vi "Add Labels.vi"(6 "Variant in":variant, 7 "Shift Pressed?":bool, 8 "error in (no error)":errorcluster, 10 "QD Combo Box Ref":refnum<vi>, 11 "QD Launch VI Ref":refnum<vi>) -> (0 "error out":errorcluster, 4 "Variant out":variant)   [LabVIEW 2017]
doc: "Add labels to SubVIs, labels to structure objects or wire labels.\n\nUsage:\nThis quick-drop plug-in works only in the block diagram.\nPress Ctrl+Space Ctrl+Q to add the labels to the selected items. If you insert a text into the combo box you will add this to the wire label.\nIf the plug-in is called using the SHIFT key than the label will be removed. \n\nDefault Shortcut - [Q]"
uses:
  8d00bab7-6807-40e1-91ac-73bbb8bf2eb0.vi
  78b8683c-1840-4b62-98b6-1b9e21eee10c.vi
panel:
  # "Do not change the connector pane of this VI.\n\nSee the block diagram for directions on how to use this template."
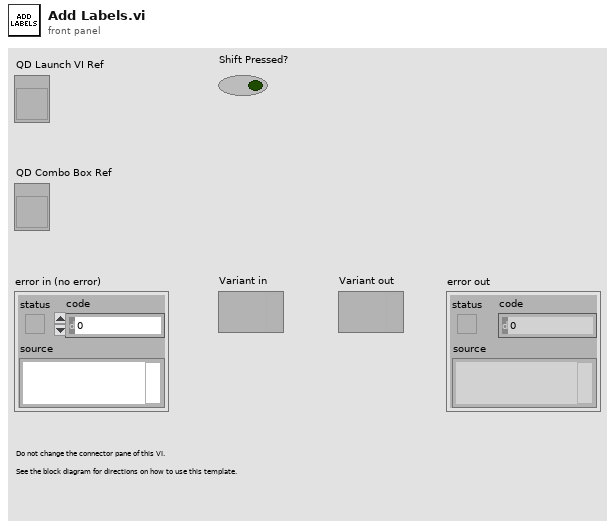
[diagram p1: front panel]
types:
  T1 = enum16{"MultiFrameStructure", "Structure", "Wire", "Constant", "FlatSequence", "Node"}
  T2 = enum16{"MultiFrameStructure", "Structure", "Wire", "Constant", "FlatSequence", "Node"}[]
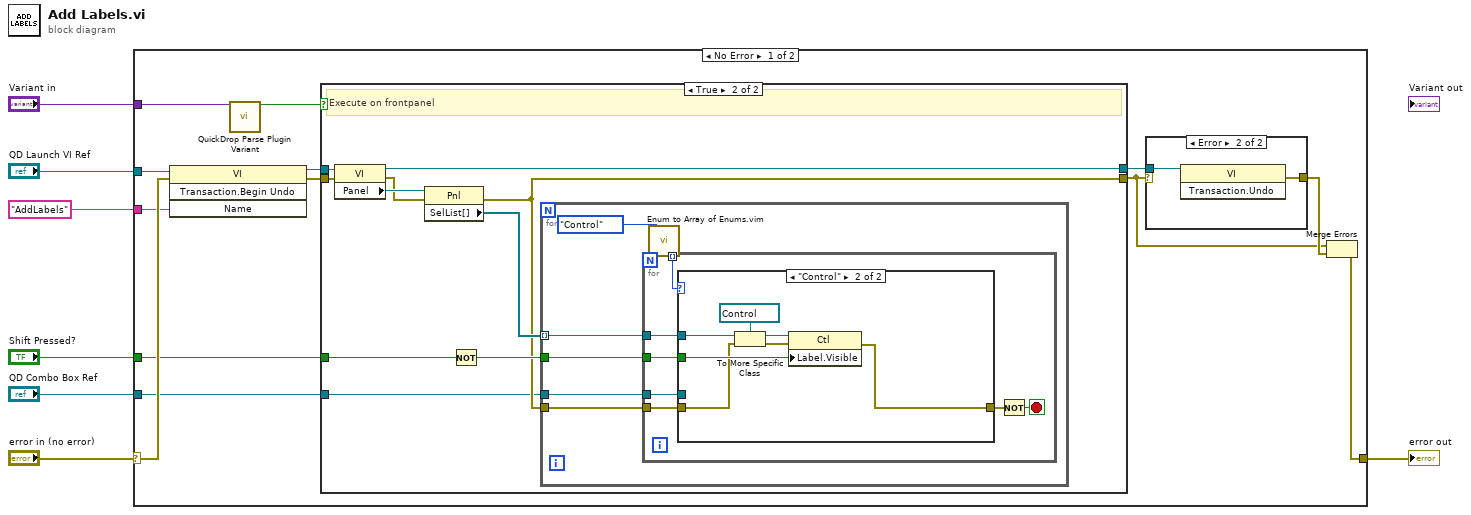
[diagram p0: block diagram]
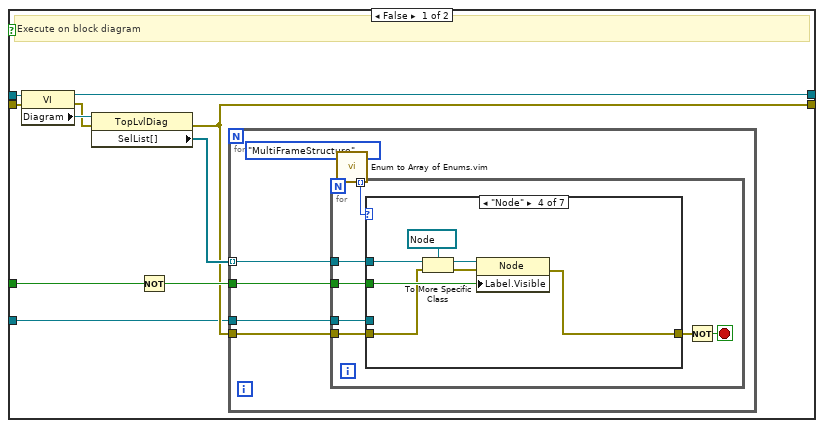
[diagram p2: hidden frame]
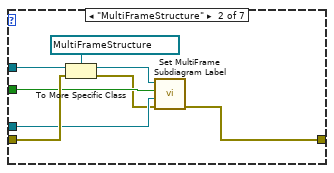
[diagram p4: hidden frame]
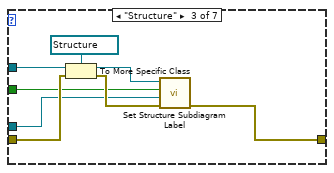
[diagram p5: hidden frame]
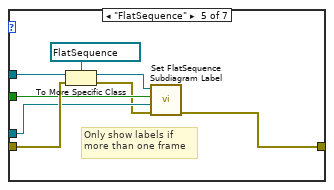
[diagram p6: hidden frame]
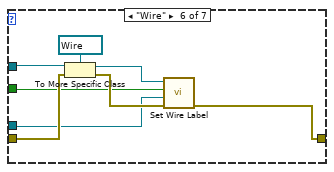
[diagram p7: hidden frame]
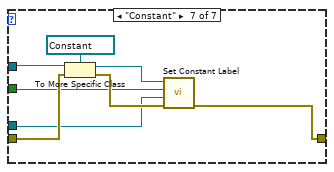
[diagram p8: hidden frame]
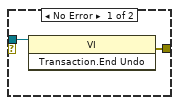
[diagram p10: hidden frame]
diagram:
  n1 = case shown="No Error" "error in (no error)" {
    selector: "error in (no error)" -> [w19 w127]
    tunnel: [w9 w127] -> w2
    tunnel: "Variant in" -> [w20 _]
    tunnel: "QD Launch VI Ref" -> [w17 _]
    tunnel: "AddLabels" ("Undo Name") -> [w18 _]
    tunnel: "Shift Pressed?" -> [w11 _]
    tunnel: "QD Combo Box Ref" -> [w10 _]
    frame No Error {
      n2 = invoke class="VI" method="Transaction.Begin Undo"(reference=w17, error in=w19, "Name"=w18) -> (reference out=w14:refnum<vi>, error out=w15:errorcluster)  [unwired: 1 in, 2 out]
      n3 = call <vilib>:"QuickDrop Parse Plugin Variant.vi"("QDKS Variant in"=w20) -> ("QD Launch VI Panel?"=w13:bool)  [unwired: 12 in, 2 out]
      n4 = case shown="True" w13 {
        tunnel: w15 -> [w30 w101]
        tunnel: w14 -> [w29 w100]
        tunnel: [w23 w94] -> w8
        tunnel: [w25 w96] -> w12
        tunnel: w11 -> [w21 w92]
        tunnel: w10 -> [w22 w93]
        frame False {
          # "Execute on block diagram"
          n5 = property class="VI"(reference=w29, error in=w30) -> (reference out=w25:refnum<vi>, error out=w26:errorcluster, "Diagram"=w28:refnum<vi>)
          n6 = property class="TopLvlDiag"(reference=w28, error in=w26) -> (error out=w23:errorcluster, "SelList[]"=w27:refnum<vi>[])  [unwired: 1 out]
          n7 = Not(x=w21) -> (.not. x?=w24:bool)
          n8 = for {
            tunnel: w27 -> [w31] mode=indexing
            tunnel: w24 -> [w32]
            tunnel: w23 -> [w33]
            tunnel: w22 -> [w34]
            n9 = call "Enum to Array of Enums.vim"("enum"=T1."MultiFrameStructure") -> ("array of enums"=w36:T2)
            n10 = for {
              tunnel: w36 -> [w43] mode=indexing
              tunnel: w33 -> [w42]
              tunnel: w32 -> [w40]
              tunnel: w31 -> [w39]
              tunnel: w34 -> [w38]
              stop <- w41 stop-if-true
              n11 = case shown="\"Node\"" w43 {
                tunnel: w42 -> [w44 w50 w58 w62 w73 w79 w88]
                tunnel: [w44 w45 w56 w61 w68 w78 w87] -> w37
                tunnel: w40 -> [_ w49 w54 w64 w71 w76 w85]
                tunnel: w39 -> [_ w51 w59 w63 w74 w80 w89]
                tunnel: w38 -> [_ w48 w53 _ w70 w77 w86]
                frame Default {
                }
                frame "MultiFrameStructure" {
                  n12 = To More Specific Class(target class=refnum<vi> refnum, reference=w51, error in=w50) -> (specific class reference=w46:refnum<vi>, error out=w47:errorcluster)
                  n13 = call "Set MultiFrame Subdiagram Label.vi"("error in (no error)"=w47, "QD Combo Box Ref"=w48, "Shift Not Pressed?"=w49, "MultiFrame in"=w46) -> ("error out"=w45:errorcluster)  [unwired: 7 in]
                }
                frame "Structure" {
                  n14 = To More Specific Class(target class=refnum<vi> refnum, reference=w59, error in=w58) -> (specific class reference=w55:refnum<vi>, error out=w57:errorcluster)
                  n15 = call "Set Structure Subdiagram Label.vi"("error in (no error)"=w57, "QD Combo Box Ref"=w53, "Shift Not Pressed?"=w54, "Structure in"=w55) -> ("error out"=w56:errorcluster)  [unwired: 7 in]
                }
                frame "Node" {
                  n16 = To More Specific Class(target class=refnum<vi> refnum, reference=w63, error in=w62) -> (specific class reference=w65:refnum<vi>, error out=w66:errorcluster)
                  n17 = property class="Node"(reference=w65, error in=w66, "Label.Visible"=w64) -> (error out=w61:errorcluster)  [unwired: 1 out]
                }
                frame "FlatSequence" {
                  # "Only show labels if\nmore than one frame"
                  n18 = To More Specific Class(target class=refnum<vi> refnum, reference=w74, error in=w73) -> (specific class reference=w72:refnum<vi>, error out=w69:errorcluster)
                  n19 = call "Set FlatSequence Subdiagram Label.vi"("error in (no error)"=w69, "QD Combo Box Ref"=w70, "Shift Not Pressed?"=w71, "FlatSequence in"=w72) -> ("error out"=w68:errorcluster)  [unwired: 7 in]
                }
                frame "Wire" {
                  n20 = To More Specific Class(target class=refnum<vi> refnum, reference=w80, error in=w79) -> (specific class reference=w82:refnum<vi>, error out=w81:errorcluster)
                  n21 = call "Set Wire Label.vi"("error in (no error)"=w81, "QD Combo Box Ref"=w77, "Shift Not Pressed?"=w76, "Wire in"=w82) -> ("error out"=w78:errorcluster)  [unwired: 7 in]
                }
                frame "Constant" {
                  n22 = To More Specific Class(target class=refnum<vi> refnum, reference=w89, error in=w88) -> (specific class reference=w84:refnum<vi>, error out=w90:errorcluster)
                  n23 = call "Set Constant Label.vi"("error in (no error)"=w90, "QD Combo Box Ref"=w86, "Shift Not Pressed?"=w85, "Constant in"=w84) -> ("error out"=w87:errorcluster)  [unwired: 7 in]
                }
              }
              n24 = Not(x=w37) -> (.not. x?=w41:bool)
            }
          }
        }
        frame True {
          # "Execute on frontpanel"
          n25 = property class="VI"(reference=w100, error in=w101) -> (reference out=w96:refnum<vi>, error out=w97:errorcluster, "Panel"=w99:refnum<vi>)
          n26 = property class="Pnl"(reference=w99, error in=w97) -> (error out=w94:errorcluster, "SelList[]"=w98:refnum<vi>[])  [unwired: 1 out]
          n27 = Not(x=w92) -> (.not. x?=w95:bool)
          n28 = for {
            tunnel: w98 -> [w102] mode=indexing
            tunnel: w95 -> [w103]
            tunnel: w94 -> [w104]
            tunnel: w93 -> [w105]
            n29 = call "Enum to Array of Enums.vim"("enum"=enum16{"Control"}."Control") -> ("array of enums"=w107:enum16{"Control"}[])
            n30 = for {
              tunnel: w107 -> [w114] mode=indexing
              tunnel: w104 -> [w113]
              tunnel: w103 -> [w111]
              tunnel: w102 -> [w110]
              tunnel: w105 -> [w109]
              stop <- w112 stop-if-true
              n31 = case shown="\"Control\"" w114 {
                tunnel: w113 -> [w115 w117]
                tunnel: [w115 w116] -> w108
                tunnel: w111 -> [_ w119]
                tunnel: w110 -> [_ w118]
                tunnel: w109 -> [_ _]
                frame Default {
                }
                frame "Control" {
                  n32 = To More Specific Class(target class=refnum<vi> refnum, reference=w118, error in=w117) -> (specific class reference=w120:refnum<vi>, error out=w121:errorcluster)
                  n33 = property class="Ctl"(reference=w120, error in=w121, "Label.Visible"=w119) -> (error out=w116:errorcluster)  [unwired: 1 out]
                }
              }
              n34 = Not(x=w108) -> (.not. x?=w112:bool)
            }
          }
        }
      }
      n35 = case shown="Error" w8 {
        tunnel: [w124 w126] -> w16
        tunnel: w12 -> [w123 w125]
        frame No Error {
          n36 = invoke class="VI" method="Transaction.End Undo"(reference=w123) -> (error out=w124:errorcluster)  [unwired: 2 in, 2 out]
        }
        frame Error {
          n37 = invoke class="VI" method="Transaction.Undo"(reference=w125) -> (error out=w126:errorcluster)  [unwired: 2 in, 2 out]
        }
      }
      n38 = Merge Errors(w8, w16) -> (w9:errorcluster)
    }
    frame Error {
    }
  }
  "error out" <- w2
